vi "GeoData.vi"() -> ()   [LabVIEW 2017] (continued)
city\tID\tFremont County\tH1\n83429\t16043\tIsland park\tID\tFremont County\tH1\n83445\t16043\tSaint anthony\tID\tFremont County\tH1\n83436\t16043\tNewdale\tID\tFremont County\tH1\n83440\t16043\tRexburg\tID\tFremont County\tH1\n83438\t16043\tParker\tID\tFremont County\tH1\n83420\t16043\tAshton\tID\tFremont County\tH1\n83451\t16043\tTeton\tID\tFremont County\tH1\n83433\t16043\tMacks inn\tID\tFremont County\tH1\n83421\t16043\tChester\tID\tFremont County\tH1\n83629\t16045\tHorseshoe bend\tID\tGem County\tH1\n83617\t16045\tEmmett\tID\tGem County\tH1\n83607\t16045\tCaldwell\tID\tGem County\tH1\n83655\t16045\tNew plymouth\tID\tGem County\tH1\n83657\t16045\tOla\tID\tGem County\tH1\n83670\t16045\tSweet\tID\tGem County\tH1\n83636\t16045\tLetha\tID\tGem County\tH1\n83616\t16045\tEagle\tID\tGem County\tH1\n83330\t16047\tGooding\tID\tGooding County\tH1\n83355\t16047\tWendell\tID\tGooding County\tH1\n83338\t16047\tJerome\tID\tGooding County\tH1\n83332\t16047\tHagerman\tID\tGooding County\tH1\n83337\t16047\tHill city\tID\tGooding County\tH1\n83316\t16047\tBuhl\tID\tGooding County\tH1\n83314\t16047\tBliss\tID\tGooding County\tH1\n83352\t16047\tShoshone\tID\tGooding County\tH1\n83549\t16049\tRiggins\tID\tIdaho County\tH1\n83539\t16049\tKooskia\tID\tIdaho County\tH1\n83547\t16049\tPollock\tID\tIdaho County\tH1\n83526\t16049\tFerdinand\tID\tIdaho County\tH1\n83525\t16049\tElk city\tID\tIdaho County\tH1\n83542\t16049\tLucile\tID\tIdaho County\tH1\n83671\t16049\tWarren\tID\tIdaho County\tH1\n83552\t16049\tStites\tID\tIdaho County\tH1\n83522\t16049\tCottonwood\tID\tIdaho County\tH1\n83554\t16049\tWhite bird\tID\tIdaho County\tH1\n83654\t16049\tNew meadows\tID\tIdaho County\tH1\n83530\t16049\tGrangeville\tID\tIdaho County\tH1\n83536\t16049\tKamiah\tID\tIdaho County\tH1\n83533\t16049\tGreencreek\tID\tIdaho County\tH1\n83434\t16051\tMenan\tID\tJefferson County\tH1\n83442\t16051\tRigby\tID\tJefferson County\tH1\n83450\t16051\tTerreton\tID\tJefferson County\tH1\n83443\t16051\tRirie\tID\tJefferson County\tH1\n83425\t16051\tHamer\tID\tJefferson County\tH1\n83444\t16051\tRoberts\tID\tJefferson County\tH1\n83401\t16051\tIdaho falls\tID\tJefferson County\tH1\n83431\t16051\tLewisville\tID\tJefferson County\tH1\n83402\t16051\tIdaho falls\tID\tJefferson County\tH1\n83435\t16051\tMonteview\tID\tJefferson County\tH1\n83325\t16053\tEden\tID\tJerome County\tH1\n83335\t16053\tHazelton\tID\tJerome County\tH1\n83338\t16053\tJerome\tID\tJerome County\tH1\n83301\t16053\tTwin falls\tID\tJerome County\tH1\n83347\t16053\tPaul\tID\tJerome County\tH1\n83810\t16055\tCataldo\tID\tKootenai County\tH1\n83876\t16055\tWorley\tID\tKootenai County\tH1\n83803\t16055\tBayview\tID\tKootenai County\tH1\n83842\t16055\tMedimont\tID\tKootenai County\tH1\n83877\t16055\tPost falls\tID\tKootenai County\tH1\n83815\t16055\tCoeur d alene\tID\tKootenai County\tH1\n83861\t16055\tSaint maries\tID\tKootenai County\tH1\n83869\t16055\tSpirit lake\tID\tKootenai County\tH1\n83816\t16055\tCoeur d alene\tID\tKootenai County\tH1\n83801\t16055\tAthol\tID\tKootenai County\tH1\n83835\t16055\tHayden\tID\tKootenai County\tH1\n83854\t16055\tPost falls\tID\tKootenai County\tH1\n83858\t16055\tRathdrum\tID\tKootenai County\tH1\n83851\t16055\tPlummer\tID\tKootenai County\tH1\n83814\t16055\tCoeur d alene\tID\tKootenai County\tH1\n83833\t16055\tHarrison\tID\tKootenai County\tH1\n83844\t16057\tMoscow\tID\tLatah County\tH1\n83535\t16057\tJuliaetta\tID\tLatah County\tH1\n83843\t16057\tMoscow\tID\tLatah County\tH1\n83823\t16057\tDeary\tID\tLatah County\tH1\n83857\t16057\tPrinceton\tID\tLatah County\tH1\n83834\t16057\tHarvard\tID\tLatah County\tH1\n83806\t16057\tBovill\tID\tLatah County\tH1\n83855\t16057\tPotlatch\tID\tLatah County\tH1\n83824\t16057\tDesmet\tID\tLatah County\tH1\n83872\t16057\tViola\tID\tLatah County\tH1\n83832\t16057\tGenesee\tID\tLatah County\tH1\n83871\t16057\tTroy\tID\tLatah County\tH1\n83537\t16057\tKendrick\tID\tLatah County\tH1\n83253\t16059\tMay\tID\tLemhi County\tH1\n83226\t16059\tChallis\tID\tLemhi County\tH1\n83462\t16059\tCarmen\tID\tLemhi County\tH1\n83469\t16059\tShoup\tID\tLemhi County\tH1\n83468\t16059\tTendoy\tID\tLemhi County\tH1\n83463\t16059\tGibbonsville\tID\tLemhi County\tH1\n83466\t16059\tNorth fork\tID\tLemhi County\tH1\n83235\t16059\tEllis\tID\tLemhi County\tH1\n83467\t16059\tSalmon\tID\tLemhi County\tH1\n83464\t16059\tLeadore\tID\tLemhi County\tH1\n83465\t16059\tLemhi\tID\tLemhi County\tH1\n83229\t16059\tCobalt\tID\tLemhi County\tH1\n83555\t16061\tWinchester\tID\tLewis County\tH1\n83544\t16061\tOrofino\tID\tLewis County\tH1\n83524\t16061\tCuldesac\tID\tLewis County\tH1\n83548\t16061\tReubens\tID\tLewis County\tH1\n83523\t16061\tCraigmont\tID\tLewis County\tH1\n83543\t16061\tNezperce\tID\tLewis County\tH1\n83545\t16061\tPeck\tID\tLewis County\tH1\n83536\t16061\tKamiah\tID\tLewis County\tH1\n83330\t16063\tGooding\tID\tLincoln County\tH1\n83327\t16063\tFairfield\tID\tLincoln County\tH1\n83349\t16063\tRichfield\tID\tLincoln County\tH1\n83324\t16063\tDietrich\tID\tLincoln County\tH1\n83352\t16063\tShoshone\tID\tLincoln County\tH1\n83347\t16063\tPaul\tID\tLincoln County\tH1\n83434\t16065\tMenan\tID\tMadison County\tH1\n83452\t16065\tTetonia\tID\tMadison County\tH1\n83422\t16065\tDriggs\tID\tMadison County\tH1\n83448\t16065\tSugar city\tID\tMadison County\tH1\n83445\t16065\tSaint anthony\tID\tMadison County\tH1\n83436\t16065\tNewdale\tID\tMadison County\tH1\n83440\t16065\tRexburg\tID\tMadison County\tH1\n83460\t16065\tRexburg\tID\tMadison County\tH1\n83451\t16065\tTeton\tID\tMadison County\tH1\n83441\t16065\tRexburg\tID\tMadison County\tH1\n83343\t16067\tMinidoka\tID\tMinidoka County\tH1\n83318\t16067\tBurley\tID\tMinidoka County\tH1\n83350\t16067\tRupert\tID\tMinidoka County\tH1\n83336\t16067\tHeyburn\tID\tMinidoka County\tH1\n83347\t16067\tPaul\tID\tMinidoka County\tH1\n83555\t16069\tWinchester\tID\tNez Perce County\tH1\n83524\t16069\tCuldesac\tID\tNez Perce County\tH1\n83535\t16069\tJuliaetta\tID\tNez Perce County\tH1\n83548\t16069\tReubens\tID\tNez Perce County\tH1\n83501\t16069\tLewiston\tID\tNez Perce County\tH1\n83545\t16069\tPeck\tID\tNez Perce County\tH1\n83540\t16069\tLapwai\tID\tNez Perce County\tH1\n83541\t16069\tLenore\tID\tNez Perce County\tH1\n83832\t16069\tGenesee\tID\tNez Perce County\tH1\n83537\t16069\tKendrick\tID\tNez Perce County\tH1\n83252\t16071\tMalad city\tID\tOneida County\tH1\n83342\t16071\tMalta\tID\tOneida County\tH1\n83243\t16071\tHolbrook\tID\tOneida County\tH1\n83639\t16073\tMarsing\tID\tOwyhee County\tH1\n83641\t16073\tMelba\tID\tOwyhee County\tH1\n83650\t16073\tMurphy\tID\tOwyhee County\tH1\n83604\t16073\tBruneau\tID\tOwyhee County\tH1\n83627\t16073\tHammett\tID\tOwyhee County\tH1\n83628\t16073\tHomedale\tID\tOwyhee County\tH1\n83624\t16073\tGrand view\tID\tOwyhee County\tH1\n83302\t16073\tRogerson\tID\tOwyhee County\tH1\n83619\t16075\tFruitland\tID\tPayette County\tH1\n83660\t16075\tParma\tID\tPayette County\tH1\n83607\t16075\tCaldwell\tID\tPayette County\tH1\n83655\t16075\tNew plymouth\tID\tPayette County\tH1\n83661\t16075\tPayette\tID\tPayette County\tH1\n83204\t16077\tPocatello\tID\tPower County\tH1\n83271\t16077\tRockland\tID\tPower County\tH1\n83211\t16077\tAmerican falls\tID\tPower County\tH1\n83212\t16077\tArbon\tID\tPower County\tH1\n83830\t16079\tFernwood\tID\tShoshone County\tH1\n83849\t16079\tOsburn\tID\tShoshone County\tH1\n83810\t16079\tCataldo\tID\tShoshone County\tH1\n83802\t16079\tAvery\tID\tShoshone County\tH1\n83868\t16079\tSmelterville\tID\tShoshone County\tH1\n83850\t16079\tPinehurst\tID\tShoshone County\tH1\n83861\t16079\tSaint maries\tID\tShoshone County\tH1\n83873\t16079\tWallace\tID\tShoshone County\tH1\n83839\t16079\tKingston\tID\tShoshone County\tH1\n83846\t16079\tMullan\tID\tShoshone County\tH1\n83837\t16079\tKellogg\tID\tShoshone County\tH1\n83867\t16079\tSilverton\tID\tShoshone County\tH1\n83808\t16079\tCalder\tID\tShoshone County\tH1\n83812\t16079\tClarkia\tID\tShoshone County\tH1\n83874\t16079\tMurray\tID\tShoshone County\tH1\n83424\t16081\tFelt\tID\tTeton County\tH1\n83452\t16081\tTetonia\tID\tTeton County\tH1\n83422\t16081\tDriggs\tID\tTeton County\tH1\n83455\t16081\tVictor\tID\tTeton County\tH1\n83436\t16081\tNewdale\tID\tTeton County\tH1\n83303\t16083\tTwin falls\tID\tTwin Falls County\tH1\n83328\t16083\tFiler\tID\tTwin Falls County\tH1\n83332\t16083\tHagerman\tID\tTwin Falls County\tH1\n83344\t16083\tMurtaugh\tID\tTwin Falls County\tH1\n83301\t16083\tTwin falls\tID\tTwin Falls County\tH1\n83321\t16083\tCastleford\tID\tTwin Falls County\tH1\n83316\t16083\tBuhl\tID\tTwin Falls County\tH1\n83341\t16083\tKimberly\tID\tTwin Falls County\tH1\n83334\t16083\tHansen\tID\tTwin Falls County\tH1\n83302\t16083\tRogerson\tID\tTwin Falls County\tH1\n83638\t16085\tMccall\tID\tValley County\tH1\n83615\t16085\tDonnelly\tID\tValley County\tH1\n83677\t16085\tYellow pine\tID\tValley County\tH1\n83611\t16085\tCascade\tID\tValley County\tH1\n83635\t16085\tLake fork\tID\tValley County\tH1\n83632\t16087\tIndian valley\tID\tWashington County\tH1\n83645\t16087\tMidvale\tID\tWashington County\tH1\n83610\t16087\tCambridge\tID\tWashington County\tH1\n83672\t16087\tWeiser\tID\tWashington County\tH1\n83661\t16087\tPayette\tID\tWashington County\tH1\n62301\t17001\tQuincy\tIL\tAdams County\tH1\n62306\t17001\tQuincy\tIL\tAdams County\tH1\n62379\t17001\tWarsaw\tIL\tAdams County\tH1\n62376\t17001\tUrsa\tIL\tAdams County\tH1\n62316\t17001\tBowen\tIL\tAdams County\tH1\n62314\t17001\tBaylis\tIL\tAdams County\tH1\n62365\t17001\tPlainville\tIL\tAdams County\tH1\n62320\t17001\tCamp point\tIL\tAdams County\tH1\n62305\t17001\tQuincy\tIL\tAdams County\tH1\n62351\t17001\tMendon\tIL\tAdams County\tH1\n62380\t17001\tWest point\tIL\tAdams County\tH1\n62324\t17001\tClayton\tIL\tAdams County\tH1\n62343\t17001\tHull\tIL\tAdams County\tH1\n62360\t17001\tPayson\tIL\tAdams County\tH1\n62312\t17001\tBarry\tIL\tAdams County\tH1\n62373\t17001\tSutter\tIL\tAdams County\tH1\n62347\t17001\tLiberty\tIL\tAdams County\tH1\n62346\t17001\tLa prairie\tIL\tAdams County\tH1\n62311\t17001\tAugusta\tIL\tAdams County\tH1\n62359\t17001\tPaloma\tIL\tAdams County\tH1\n62348\t17001\tLima\tIL\tAdams County\tH1\n62339\t17001\tGolden\tIL\tAdams County\tH1\n62349\t17001\tLoraine\tIL\tAdams County\tH1\n62338\t17001\tFowler\tIL\tAdams County\tH1\n62325\t17001\tCoatsburg\tIL\tAdams County\tH1\n62914\t17003\tCairo\tIL\tAlexander County\tH1\n62962\t17003\tMiller city\tIL\tAlexander County\tH1\n62952\t17003\tJonesboro\tIL\tAlexander County\tH1\n62957\t17003\tMc clure\tIL\tAlexander County\tH1\n62969\t17003\tOlive branch\tIL\tAlexander County\tH1\n62990\t17003\tThebes\tIL\tAlexander County\tH1\n62992\t17003\tUllin\tIL\tAlexander County\tH1\n62993\t17003\tUnity\tIL\tAlexander County\tH1\n62988\t17003\tTamms\tIL\tAlexander County\tH1\n62249\t17005\tHighland\tIL\tBond County\tH1\n62231\t17005\tCarlyle\tIL\tBond County\tH1\n62275\t17005\tPocahontas\tIL\tBond County\tH1\n62019\t17005\tDonnellson\tIL\tBond County\tH1\n62253\t17005\tKeyesport\tIL\tBond County\tH1\n62262\t17005\tMulberry grove\tIL\tBond County\tH1\n62017\t17005\tCoffeen\tIL\tBond County\tH1\n62086\t17005\tSorento\tIL\tBond County\tH1\n62074\t17005\tNew douglas\tIL\tBond County\tH1\n62284\t17005\tSmithboro\tIL\tBond County\tH1\n62246\t17005\tGreenville\tIL\tBond County\tH1\n61114\t17007\tRockford\tIL\tBoone County\tH1\n60152\t17007\tMarengo\tIL\tBoone County\tH1\n61011\t17007\tCaledonia\tIL\tBoone County\tH1\n61012\t17007\tCapron\tIL\tBoone County\tH1\n61008\t17007\tBelvidere\tIL\tBoone County\tH1\n61073\t17007\tRoscoe\tIL\tBoone County\tH1\n61080\t17007\tSouth beloit\tIL\tBoone County\tH1\n61038\t17007\tGarden prairie\tIL\tBoone County\tH1\n61111\t17007\tLoves park\tIL\tBoone County\tH1\n60033\t17007\tHarvard\tIL\tBoone County\tH1\n60145\t17007\tKingston\tIL\tBoone County\tH1\n61065\t17007\tPoplar grove\tIL\tBoone County\tH1\n61107\t17007\tRockford\tIL\tBoone County\tH1\n61108\t17007\tRockford\tIL\tBoone County\tH1\n60135\t17007\tGenoa\tIL\tBoone County\tH1\n60146\t17007\tKirkland\tIL\tBoone County\tH1\n61016\t17007\tCherry valley\tIL\tBoone County\tH1\n62375\t17009\tTimewell\tIL\tBrown County\tH1\n62314\t17009\tBaylis\tIL\tBrown County\tH1\n62353\t17009\tMount sterling\tIL\tBrown County\tH1\n62378\t17009\tVersailles\tIL\tBrown County\tH1\n61560\t17011\tPutnam\tIL\tBureau County\tH1\n61338\t17011\tManlius\tIL\tBureau County\tH1\n61421\t17011\tBradford\tIL\tBureau County\tH1\n61337\t17011\tMalden\tIL\tBureau County\tH1\n61349\t17011\tOhio\tIL\tBureau County\tH1\n61314\t17011\tBuda\tIL\tBureau County\tH1\n61443\t17011\tKewanee\tIL\tBureau County\tH1\n61342\t17011\tMendota\tIL\tBureau County\tH1\n61379\t17011\tWyanet\tIL\tBureau County\tH1\n61312\t17011\tArlington\tIL\tBureau County\tH1\n61344\t17011\tMineral\tIL\tBureau County\tH1\n61346\t17011\tNew bedford\tIL\tBureau County\tH1\n61283\t17011\tTampico\tIL\tBureau County\tH1\n61356\t17011\tPrinceton\tIL\tBureau County\tH1\n61374\t17011\tVan orin\tIL\tBureau County\tH1\n61243\t17011\tDeer grove\tIL\tBureau County\tH1\n61354\t17011\tPeru\tIL\tBureau County\tH1\n61362\t17011\tSpring valley\tIL\tBureau County\tH1\n61368\t17011\tTiskilwa\tIL\tBureau County\tH1\n61376\t17011\tWalnut\tIL\tBureau County\tH1\n61315\t17011\tBureau\tIL\tBureau County\tH1\n61361\t17011\tSheffield\tIL\tBureau County\tH1\n61345\t17011\tNeponset\tIL\tBureau County\tH1\n61320\t17011\tDalzell\tIL\tBureau County\tH1\n61317\t17011\tCherry\tIL\tBureau County\tH1\n61329\t17011\tLadd\tIL\tBureau County\tH1\n61330\t17011\tLa moille\tIL\tBureau County\tH1\n61359\t17011\tSeatonville\tIL\tBureau County\tH1\n61323\t17011\tDover\tIL\tBureau County\tH1\n61328\t17011\tKasbeer\tIL\tBureau County\tH1\n61234\t17011\tAnnawan\tIL\tBureau County\tH1\n61322\t17011\tDepue\tIL\tBureau County\tH1\n62047\t17013\tHardin\tIL\tCalhoun County\tH1\n62070\t17013\tMozier\tIL\tCalhoun County\tH1\n62053\t17013\tKampsville\tIL\tCalhoun County\tH1\n62006\t17013\tBatchtown\tIL\tCalhoun County\tH1\n62045\t17013\tHamburg\tIL\tCalhoun County\tH1\n62036\t17013\tGolden eagle\tIL\tCalhoun County\tH1\n62355\t17013\tNebo\tIL\tCalhoun County\tH1\n62065\t17013\tMichael\tIL\tCalhoun County\tH1\n62013\t17013\tBrussels\tIL\tCalhoun County\tH1\n61053\t17015\tMount carroll\tIL\tCarroll County\tH1\n61062\t17015\tPearl city\tIL\tCarroll County\tH1\n61285\t17015\tThomson\tIL\tCarroll County\tH1\n61051\t17015\tMilledgeville\tIL\tCarroll County\tH1\n61064\t17015\tPolo\tIL\tCarroll County\tH1\n61252\t17015\tFulton\tIL\tCarroll County\tH1\n61028\t17015\tElizabeth\tIL\tCarroll County\tH1\n61074\t17015\tSavanna\tIL\tCarroll County\tH1\n61270\t17015\tMorrison\tIL\tCarroll County\tH1\n61046\t17015\tLanark\tIL\tCarroll County\tH1\n61078\t17015\tShannon\tIL\tCarroll County\tH1\n61014\t17015\tChadwick\tIL\tCarroll County\tH1\n62627\t17017\tChandlerville\tIL\tCass County\tH1\n62665\t17017\tMeredosia\tIL\tCass County\tH1\n62677\t17017\tPleasant plains\tIL\tCass County\tH1\n62612\t17017\tAshland\tIL\tCass County\tH1\n62618\t17017\tBeardstown\tIL\tCass County\tH1\n62691\t17017\tVirginia\tIL\tCass County\tH1\n62673\t17017\tOakford\tIL\tCass County\tH1\n62675\t17017\tPetersburg\tIL\tCass County\tH1\n62611\t17017\tArenzville\tIL\tCass County\tH1\n62622\t17017\tBluff springs\tIL\tCass County\tH1\n61864\t17019\tPhilo\tIL\tChampaign County\tH1\n60949\t17019\tLudlow\tIL\tChampaign County\tH1\n60957\t17019\tPaxton\tIL\tChampaign County\tH1\n61802\t17019\tUrbana\tIL\tChampaign County\tH1\n61859\t17019\tOgden\tIL\tChampaign County\tH1\n61862\t17019\tPenfield\tIL\tChampaign County\tH1\n61872\t17019\tSadorus\tIL\tChampaign County\tH1\n61852\t17019\tLongview\tIL\tChampaign County\tH1\n61856\t17019\tMonticello\tIL\tChampaign County\tH1\n61878\t17019\tThomasboro\tIL\tChampaign County\tH1\n61843\t17019\tFisher\tIL\tChampaign County\tH1\n61884\t17019\tWhite heath\tIL\tChampaign County\tH1\n61851\t17019\tIvesdale\tIL\tChampaign County\tH1\n60936\t17019\tGibson city\tIL\tChampaign County\tH1\n61956\t17019\tVilla grove\tIL\tChampaign County\tH1\n61863\t17019\tPesotum\tIL\tChampaign County\tH1\n60960\t17019\tRankin\tIL\tChampaign County\tH1\n61849\t17019\tHomer\tIL\tChampaign County\tH1\n61880\t17019\tTolono\tIL\tChampaign County\tH1\n61866\t17019\tRantoul\tIL\tChampaign County\tH1\n61847\t17019\tGifford\tIL\tChampaign County\tH1\n61825\t17019\tChampaign\tIL\tChampaign County\tH1\n61822\t17019\tChampaign\tIL\tChampaign County\tH1\n61815\t17019\tBondville\tIL\tChampaign County\tH1\n61853\t17019\tMahomet\tIL\tChampaign County\tH1\n61953\t17019\tTuscola\tIL\tChampaign County\tH1\n61854\t17019\tMansfield\tIL\tChampaign County\tH1\n61810\t17019\tAllerton\tIL\tChampaign County\tH1\n61801\t17019\tUrbana\tIL\tChampaign County\tH1\n61821\t17019\tChampaign\tIL\tChampaign County\tH1\n61826\t17019\tChampaign\tIL\tChampaign County\tH1\n61873\t17019\tSaint joseph\tIL\tChampaign County\tH1\n61840\t17019\tDewey\tIL\tChampaign County\tH1\n61871\t17019\tRoyal\tIL\tChampaign County\tH1\n61845\t17019\tFoosland\tIL\tChampaign County\tH1\n61824\t17019\tChampaign\tIL\tChampaign County\tH1\n61820\t17019\tChampaign\tIL\tChampaign County\tH1\n61874\t17019\tSavoy\tIL\tChampaign County\tH1\n61875\t17019\tSeymour\tIL\tChampaign County\tH1\n61877\t17019\tSidney\tIL\tChampaign County\tH1\n61816\t17019\tBroadlands\tIL\tChampaign County\tH1\n61803\t17019\tUrbana\tIL\tChampaign County\tH1\n62545\t17021\tMechanicsburg\tIL\tChristian County\tH1\n62510\t17021\tAssumption\tIL\tChristian County\tH1\n62556\t17021\tPalmer\tIL\tChristian County\tH1\n62547\t17021\tMount auburn\tIL\tChristian County\tH1\n62555\t17021\tOwaneco\tIL\tChristian County\tH1\n62083\t17021\tRosamond\tIL\tChristian County\tH1\n62558\t17021\tPawnee\tIL\tChristian County\tH1\n62557\t17021\tPana\tIL\tChristian County\tH1\n62546\t17021\tMorrisonville\tIL\tChristian County\tH1\n62567\t17021\tStonington\tIL\tChristian County\tH1\n62568\t17021\tTaylorville\tIL\tChristian County\tH1\n62075\t17021\tNokomis\tIL\tChristian County\tH1\n62540\t17021\tKincaid\tIL\tChristian County\tH1\n62531\t17021\tEdinburg\tIL\tChristian County\tH1\n62538\t17021\tHarvel\tIL\tChristian County\tH1\n62513\t17021\tBlue mound\tIL\tChristian County\tH1\n62563\t17021\tRochester\tIL\tChristian County\tH1\n62550\t17021\tMoweaqua\tIL\tChristian County\tH1\n62570\t17021\tTovey\tIL\tChristian County\tH1\n62517\t17021\tBulpitt\tIL\tChristian County\tH1\n62478\t17023\tWest york\tIL\tClark County\tH1\n61933\t17023\tKansas\tIL\tClark County\tH1\n61944\t17023\tParis\tIL\tClark County\tH1\n62420\t17023\tCasey\tIL\tClark County\tH1\n62441\t17023\tMarshall\tIL\tClark County\tH1\n62481\t17023\tYale\tIL\tClark County\tH1\n61912\t17023\tAshmore\tIL\tClark County\tH1\n62413\t17023\tAnnapolis\tIL\tClark County\tH1\n62449\t17023\tOblong\tIL\tClark County\tH1\n62442\t17023\tMartinsville\tIL\tClark County\tH1\n62474\t17023\tWestfield\tIL\tClark County\tH1\n62423\t17023\tDennison\tIL\tClark County\tH1\n62477\t17023\tWest union\tIL\tClark County\tH1\n62448\t17025\tNewton\tIL\tClay County\tH1\n62426\t17025\tEdgewood\tIL\tClay County\tH1\n62858\t17025\tLouisville\tIL\tClay County\tH1\n62899\t17025\tXenia\tIL\tClay County\tH1\n62838\t17025\tFarina\tIL\tClay County\tH1\n62839\t17025\tFlora\tIL\tClay County\tH1\n62868\t17025\tNoble\tIL\tClay County\tH1\n62879\t17025\tSailor springs\tIL\tClay County\tH1\n62443\t17025\tMason\tIL\tClay County\tH1\n62424\t17025\tDieterich\tIL\tClay County\tH1\n62824\t17025\tClay city\tIL\tClay County\tH1\n62854\t17025\tKinmundy\tIL\tClay County\tH1\n62434\t17025\tIngraham\tIL\tClay County\tH1\n62249\t17027\tHighland\tIL\tClinton County\tH1\n62231\t17027\tCarlyle\tIL\tClinton County\tH1\n62275\t17027\tPocahontas\tIL\tClinton County\tH1\n62219\t17027\tBeckemeyer\tIL\tClinton County\tH1\n62882\t17027\tSandoval\tIL\tClinton County\tH1\n62253\t17027\tKeyesport\tIL\tClinton County\tH1\n62252\t17027\tHuey\tIL\tClinton County\tH1\n62250\t17027\tHoffman\tIL\tClinton County\tH1\n62266\t17027\tNew memphis\tIL\tClinton County\tH1\n62215\t17027\tAlbers\tIL\tClinton County\tH1\n62801\t17027\tCentralia\tIL\tClinton County\tH1\n62875\t17027\tPatoka\tIL\tClinton County\tH1\n62216\t17027\tAviston\tIL\tClinton County\tH1\n62230\t17027\tBreese\tIL\tClinton County\tH1\n62265\t17027\tNew baden\tIL\tClinton County\tH1\n62218\t17027\tBartelso\tIL\tClinton County\tH1\n62245\t17027\tGermantown\tIL\tClinton County\tH1\n62246\t17027\tGreenville\tIL\tClinton County\tH1\n62258\t17027\tMascoutah\tIL\tClinton County\tH1\n62293\t17027\tTrenton\tIL\tClinton County\tH1\n62447\t17029\tNeoga\tIL\tColes County\tH1\n61920\t17029\tCharleston\tIL\tColes County\tH1\n62469\t17029\tTrilla\tIL\tColes County\tH1\n62440\t17029\tLerna\tIL\tColes County\tH1\n61931\t17029\tHumboldt\tIL\tColes County\tH1\n62420\t17029\tCasey\tIL\tColes County\tH1\n61943\t17029\tOakland\tIL\tColes County\tH1\n61911\t17029\tArthur\tIL\tColes County\tH1\n61930\t17029\tHindsboro\tIL\tColes County\tH1\n61912\t17029\tAshmore\tIL\tColes County\tH1\n61910\t17029\tArcola\tIL\tColes County\tH1\n61938\t17029\tMattoon\tIL\tColes County\tH1\n61951\t17029\tSullivan\tIL\tColes County\tH1\n61928\t17029\tGays\tIL\tColes County\tH1\n62474\t17029\tWestfield\tIL\tColes County\tH1\n60067\t17031\tPalatine\tIL\tCook County\tH1\n60056\t17031\tMount prospect\tIL\tCook County\tH1\n60029\t17031\tGolf\tIL\tCook County\tH1\n60305\t17031\tRiver forest\tIL\tCook County\tH1\n60417\t17031\tCrete\tIL\tCook County\tH1\n60422\t17031\tFlossmoor\tIL\tCook County\tH1\n60462\t17031\tOrland park\tIL\tCook County\tH1\n60455\t17031\tBridgeview\tIL\tCook County\tH1\n60456\t17031\tHometown\tIL\tCook County\tH1\n60463\t17031\tPalos heights\tIL\tCook County\tH1\n60525\t17031\tLa grange\tIL\tCook County\tH1\n60162\t17031\tHillside\tIL\tCook County\tH1\n60619\t17031\tChicago\tIL\tCook County\tH1\n60654\t17031\tChicago\tIL\tCook County\tH1\n60632\t17031\tChicago\tIL\tCook County\tH1\n60682\t17031\tChicago\tIL\tCook County\tH1\n60689\t17031\tChicago\tIL\tCook County\tH1\n60684\t17031\tChicago\tIL\tCook County\tH1\n60669\t17031\tChicago\tIL\tCook County\tH1\n60068\t17031\tPark ridge\tIL\tCook County\tH1\n60090\t17031\tWheeling\tIL\tCook County\tH1\n60091\t17031\tWilmette\tIL\tCook County\tH1\n60089\t17031\tBuffalo grove\tIL\tCook County\tH1\n60053\t17031\tMorton grove\tIL\tCook County\tH1\n60203\t17031\tEvanston\tIL\tCook County\tH1\n60192\t17031\tHoffman estates\tIL\tCook County\tH1\n60402\t17031\tBerwyn\tIL\tCook County\tH1\n60303\t17031\tOak park\tIL\tCook County\tH1\n60172\t17031\tRoselle\tIL\tCook County\tH1\n60195\t17031\tSchaumburg\tIL\tCook County\tH1\n60176\t17031\tSchiller park\tIL\tCook County\tH1\n60439\t17031\tLemont\tIL\tCook County\tH1\n60423\t17031\tFrankfort\tIL\tCook County\tH1\n60457\t17031\tHickory hills\tIL\tCook County\tH1\n60523\t17031\tOak brook\tIL\tCook County\tH1\n60480\t17031\tWillow springs\tIL\tCook County\tH1\n60163\t17031\tBerkeley\tIL\tCook County\tH1\n60558\t17031\tWestern springs\tIL\tCook County\tH1\n60615\t17031\tChicago\tIL\tCook County\tH1\n60616\t17031\tChicago\tIL\tCook County\tH1\n60608\t17031\tChicago\tIL\tCook County\tH1\n60620\t17031\tChicago\tIL\tCook County\tH1\n60651\t17031\tChicago\tIL\tCook County\tH1\n60659\t17031\tChicago\tIL\tCook County\tH1\n60706\t17031\tHarwood heights\tIL\tCook County\tH1\n60653\t17031\tChicago\tIL\tCook County\tH1\n60639\t17031\tChicago\tIL\tCook County\tH1\n60624\t17031\tChicago\tIL\tCook County\tH1\n60647\t17031\tChicago\tIL\tCook County\tH1\n60011\t17031\tBarrington\tIL\tCook County\tH1\n60690\t17031\tChicago\tIL\tCook County\tH1\n60006\t17031\tArlington heights\tIL\tCook County\tH1\n60695\t17031\tChicago\tIL\tCook County\tH1\n60687\t17031\tChicago\tIL\tCook County\tH1\n60678\t17031\tChicago\tIL\tCook County\tH1\n60685\t17031\tChicago\tIL\tCook County\tH1\n60196\t17031\tSchaumburg\tIL\tCook County\tH1\n60070\t17031\tProspect heights\tIL\tCook County\tH1\n60026\t17031\tGlenview\tIL\tCook County\tH1\n60008\t17031\tRolling meadows\tIL\tCook County\tH1\n60301\t17031\tOak park\tIL\tCook County\tH1\n60411\t17031\tChicago heights\tIL\tCook County\tH1\n60415\t17031\tChicago ridge\tIL\tCook County\tH1\n60169\t17031\tHoffman estates\tIL\tCook County\tH1\n60438\t17031\tLansing\tIL\tCook County\tH1\n60428\t17031\tMarkham\tIL\tCook County\tH1\n60458\t17031\tJustice\tIL\tCook County\tH1\n60425\t17031\tGlenwood\tIL\tCook County\tH1\n60418\t17031\tCrestwood\tIL\tCook County\tH1\n60513\t17031\tBrookfield\tIL\tCook County\tH1\n60501\t17031\tSummit argo\tIL\tCook County\tH1\n60103\t17031\tBartlett\tIL\tCook County\tH1\n60102\t17031\tAlgonquin\tIL\tCook County\tH1\n60154\t17031\tWestchester\tIL\tCook County\tH1\n60155\t17031\tBroadview\tIL\tCook County\tH1\n60609\t17031\tChicago\tIL\tCook County\tH1\n60803\t17031\tAlsip\tIL\tCook County\tH1\n60675\t17031\tChicago\tIL\tCook County\tH1\n60633\t17031\tChicago\tIL\tCook County\tH1\n60634\t17031\tChicago\tIL\tCook County\tH1\n60645\t17031\tChicago\tIL\tCook County\tH1\n60208\t17031\tEvanston\tIL\tCook County\tH1\n60699\t17031\tChicago\tIL\tCook County\tH1\n60038\t17031\tPalatine\tIL\tCook County\tH1\n60668\t17031\tChicago\tIL\tCook County\tH1\n60701\t17031\tChicago\tIL\tCook County\tH1\n60062\t17031\tNorthbrook\tIL\tCook County\tH1\n60016\t17031\tDes plaines\tIL\tCook County\tH1\n60015\t17031\tDeerfield\tIL\tCook County\tH1\n60018\t17031\tDes plaines\tIL\tCook County\tH1\n60043\t17031\tKenilworth\tIL\tCook County\tH1\n60409\t17031\tCalumet city\tIL\tCook County\tH1\n60443\t17031\tMatteson\tIL\tCook County\tH1\n60465\t17031\tPalos hills\tIL\tCook County\tH1\n60469\t17031\tPosen\tIL\tCook County\tH1\n60471\t17031\tRichton park\tIL\tCook County\tH1\n60131\t17031\tFranklin park\tIL\tCook County\tH1\n60153\t17031\tMaywood\tIL\tCook County\tH1\n60613\t17031\tChicago\tIL\tCook County\tH1\n60622\t17031\tChicago\tIL\tCook County\tH1\n60804\t17031\tCicero\tIL\tCook County\tH1\n60649\t17031\tChicago\tIL\tCook County\tH1\n60652\t17031\tChicago\tIL\tCook County\tH1\n60631\t17031\tChicago\tIL\tCook County\tH1\n60640\t17031\tChicago\tIL\tCook County\tH1\n60626\t17031\tChicago\tIL\tCook County\tH1\n60630\t17031\tChicago\tIL\tCook County\tH1\n60636\t17031\tChicago\tIL\tCook County\tH1\n60643\t17031\tChicago\tIL\tCook County\tH1\n60499\t17031\tBedford park\tIL\tCook County\tH1\n60082\t17031\tTechny\tIL\tCook County\tH1\n60076\t17031\tSkokie\tIL\tCook County\tH1\n60202\t17031\tEvanston\tIL\tCook County\tH1\n60093\t17031\tWinnetka\tIL\tCook County\tH1\n60005\t17031\tArlington heights\tIL\tCook County\tH1\n60194\t17031\tSchaumburg\tIL\tCook County\tH1\n60302\t17031\tOak park\tIL\tCook County\tH1\n60164\t17031\tMelrose park\tIL\tCook County\tH1\n60448\t17031\tMokena\tIL\tCook County\tH1\n60453\t17031\tOak lawn\tIL\tCook County\tH1\n60459\t17031\tBurbank\tIL\tCook County\tH1\n60487\t17031\tTinley park\tIL\tCook County\tH1\n60466\t17031\tPark forest\tIL\tCook County\tH1\n60120\t17031\tElgin\tIL\tCook County\tH1\n60546\t17031\tRiverside\tIL\tCook County\tH1\n60605\t17031\tChicago\tIL\tCook County\tH1\n60607\t17031\tChicago\tIL\tCook County\tH1\n60612\t17031\tChicago\tIL\tCook County\tH1\n60621\t17031\tChicago\tIL\tCook County\tH1\n60657\t17031\tChicago\tIL\tCook County\tH1\n60655\t17031\tChicago\tIL\tCook County\tH1\n60629\t17031\tChicago\tIL\tCook County\tH1\n60637\t17031\tChicago\tIL\tCook County\tH1\n60641\t17031\tChicago\tIL\tCook County\tH1\n60625\t17031\tChicago\tIL\tCook County\tH1\n60646\t17031\tChicago\tIL\tCook County\tH1\n60602\t17031\tChicago\tIL\tCook County\tH1\n60159\t17031\tSchaumburg\tIL\tCook County\tH1\n60673\t17031\tChicago\tIL\tCook County\tH1\n60694\t17031\tChicago\tIL\tCook County\tH1\n60095\t17031\tPalatine\tIL\tCook County\tH1\n60055\t17031\tPalatine\tIL\tCook County\tH1\n60670\t17031\tChicago\tIL\tCook County\tH1\n60077\t17031\tSkokie\tIL\tCook County\tH1\n60201\t17031\tEvanston\tIL\tCook County\tH1\n60204\t17031\tEvanston\tIL\tCook County\tH1\n60010\t17031\tBarrington\tIL\tCook County\tH1\n60007\t17031\tElk grove village\tIL\tCook County\tH1\n60304\t17031\tOak park\tIL\tCook County\tH1\n60419\t17031\tDolton\tIL\tCook County\tH1\n60445\t17031\tMidlothian\tIL\tCook County\tH1\n60452\t17031\tOak forest\tIL\tCook County\tH1\n60521\t17031\tHinsdale\tIL\tCook County\tH1\n60527\t17031\tWillowbrook\tIL\tCook County\tH1\n60472\t17031\tRobbins\tIL\tCook County\tH1\n60141\t17031\tHines\tIL\tCook County\tH1\n60130\t17031\tForest park\tIL\tCook County\tH1\n60107\t17031\tStreamwood\tIL\tCook County\tH1\n60160\t17031\tMelrose park\tIL\tCook County\tH1\n60610\t17031\tChicago\tIL\tCook County\tH1\n60603\t17031\tChicago\tIL\tCook County\tH1\n60827\t17031\tRiverdale\tIL\tCook County\tH1\n60714\t17031\tNiles\tIL\tCook County\tH1\n60656\t17031\tChicago\tIL\tCook County\tH1\n60476\t17031\tThornton\tIL\tCook County\tH1\n60078\t17031\tPalatine\tIL\tCook County\tH1\n60666\t17031\tChicago\tIL\tCook County\tH1\n60454\t17031\tOak lawn\tIL\tCook County\tH1\n60065\t17031\tNorthbrook\tIL\tCook County\tH1\n60697\t17031\tChicago\tIL\tCook County\tH1\n60074\t17031\tPalatine\tIL\tCook County\tH1\n60022\t17031\tGlencoe\tIL\tCook County\tH1\n60004\t17031\tArlington heights\tIL\tCook County\tH1\n60025\t17031\tGlenview\tIL\tCook County\tH1\n60193\t17031\tSchaumburg\tIL\tCook County\tH1\n60173\t17031\tSchaumburg\tIL\tCook County\tH1\n60406\t17031\tBlue island\tIL\tCook County\tH1\n60412\t17031\tChicago heights\tIL\tCook County\tH1\n60449\t17031\tMonee\tIL\tCook County\tH1\n60426\t17031\tHarvey\tIL\tCook County\tH1\n60430\t17031\tHomewood\tIL\tCook County\tH1\n60477\t17031\tTinley park\tIL\tCook County\tH1\n60482\t17031\tWorth\tIL\tCook County\tH1\n60473\t17031\tSouth holland\tIL\tCook County\tH1\n60478\t17031\tCountry club hills\tIL\tCook County\tH1\n60526\t17031\tLa grange park\tIL\tCook County\tH1\n60484\t17031\tUniversity park\tIL\tCook County\tH1\n60534\t17031\tLyons\tIL\tCook County\tH1\n60618\t17031\tChicago\tIL\tCook County\tH1\n60604\t17031\tChicago\tIL\tCook County\tH1\n60606\t17031\tChicago\tIL\tCook County\tH1\n60617\t17031\tChicago\tIL\tCook County\tH1\n60660\t17031\tChicago\tIL\tCook County\tH1\n60661\t17031\tChicago\tIL\tCook County\tH1\n60712\t17031\tLincolnwood\tIL\tCook County\tH1\n60805\t17031\tEvergreen park\tIL\tCook County\tH1\n60674\t17031\tChicago\tIL\tCook County\tH1\n60628\t17031\tChicago\tIL\tCook County\tH1\n60623\t17031\tChicago\tIL\tCook County\tH1\n60677\t17031\tChicago\tIL\tCook County\tH1\n60681\t17031\tChicago\tIL\tCook County\tH1\n60688\t17031\tChicago\tIL\tCook County\tH1\n60017\t17031\tDes plaines\tIL\tCook County\tH1\n60171\t17031\tRiver grove\tIL\tCook County\tH1\n60165\t17031\tStone park\tIL\tCook County\tH1\n60429\t17031\tHazel crest\tIL\tCook County\tH1\n60461\t17031\tOlympia fields\tIL\tCook County\tH1\n60491\t17031\tHomer glen\tIL\tCook County\tH1\n60464\t17031\tPalos park\tIL\tCook County\tH1\n60467\t17031\tOrland park\tIL\tCook County\tH1\n60475\t17031\tSteger\tIL\tCook County\tH1\n60126\t17031\tElmhurst\tIL\tCook County\tH1\n60133\t17031\tHanover park\tIL\tCook County\tH1\n60104\t17031\tBellwood\tIL\tCook County\tH1\n60118\t17031\tDundee\tIL\tCook County\tH1\n60611\t17031\tChicago\tIL\tCook County\tH1\n60614\t17031\tChicago\tIL\tCook County\tH1\n60707\t17031\tElmwood park\tIL\tCook County\tH1\n60638\t17031\tChicago\tIL\tCook County\tH1\n60642\t17031\tChicago\tIL\tCook County\tH1\n60644\t17031\tChicago\tIL\tCook County\tH1\n60601\t17031\tChicago\tIL\tCook County\tH1\n60161\t17031\tMelrose park\tIL\tCook County\tH1\n60686\t17031\tChicago\tIL\tCook County\tH1\n60009\t17031\tElk grove village\tIL\tCook County\tH1\n60693\t17031\tChicago\tIL\tCook County\tH1\n60168\t17031\tSchaumburg\tIL\tCook County\tH1\n60179\t17031\tHoffman estates\tIL\tCook County\tH1\n62466\t17033\tSumner\tIL\tCrawford County\tH1\n62478\t17033\tWest york\tIL\tCrawford County\tH1\n62433\t17033\tHutsonville\tIL\tCrawford County\tH1\n62454\t17033\tRobinson\tIL\tCrawford County\tH1\n62451\t17033\tPalestine\tIL\tCrawford County\tH1\n62421\t17033\tClaremont\tIL\tCrawford County\tH1\n62464\t17033\tStoy\tIL\tCrawford County\tH1\n62413\t17033\tAnnapolis\tIL\tCrawford County\tH1\n62427\t17033\tFlat rock\tIL\tCrawford County\tH1\n62449\t17033\tOblong\tIL\tCrawford County\tH1\n62442\t17033\tMartinsville\tIL\tCrawford County\tH1\n62447\t17035\tNeoga\tIL\tCumberland County\tH1\n61920\t17035\tCharleston\tIL\tCumberland County\tH1\n62469\t17035\tTrilla\tIL\tCumberland County\tH1\n62440\t17035\tLerna\tIL\tCumberland County\tH1\n62445\t17035\tMontrose\tIL\tCumberland County\tH1\n62420\t17035\tCasey\tIL\tCumberland County\tH1\n62428\t17035\tGreenup\tIL\tCumberland County\tH1\n62468\t17035\tToledo\tIL\tCumberland County\tH1\n62432\t17035\tHidalgo\tIL\tCumberland County\tH1\n62462\t17035\tSigel\tIL\tCumberland County\tH1\n62436\t17035\tJewett\tIL\tCumberland County\tH1\n61938\t17035\tMattoon\tIL\tCumberland County\tH1\n62467\t17035\tTeutopolis\tIL\tCumberland County\tH1\n60152\t17037\tMarengo\tIL\tDeKalb County\tH1\n60553\t17037\tSteward\tIL\tDeKalb County\tH1\n60112\t17037\tCortland\tIL\tDeKalb County\tH1\n60552\t17037\tSomonauk\tIL\tDeKalb County\tH1\n60548\t17037\tSandwich\tIL\tDeKalb County\tH1\n61068\t17037\tRochelle\tIL\tDeKalb County\tH1\n60178\t17037\tSycamore\tIL\tDeKalb County\tH1\n60531\t17037\tLeland\tIL\tDeKalb County\tH1\n60111\t17037\tClare\tIL\tDeKalb County\tH1\n60115\t17037\tDekalb\tIL\tDeKalb County\tH1\n61052\t17037\tMonroe center\tIL\tDeKalb County\tH1\n60511\t17037\tBig rock\tIL\tDeKalb County\tH1\n60119\t17037\tElburn\tIL\tDeKalb County\tH1\n60145\t17037\tKingston\tIL\tDeKalb County\tH1\n60530\t17037\tLee\tIL\tDeKalb County\tH1\n60556\t17037\tWaterman\tIL\tDeKalb County\tH1\n60550\t17037\tShabbona\tIL\tDeKalb County\tH1\n60520\t17037\tHinckley\tIL\tDeKalb County\tH1\n60135\t17037\tGenoa\tIL\tDeKalb County\tH1\n60146\t17037\tKirkland\tIL\tDeKalb County\tH1\n60150\t17037\tMalta\tIL\tDeKalb County\tH1\n60518\t17037\tEarlville\tIL\tDeKalb County\tH1\n60140\t17037\tHampshire\tIL\tDeKalb County\tH1\n60151\t17037\tMaple park\tIL\tDeKalb County\tH1\n60129\t17037\tEsmond\tIL\tDeKalb County\tH1\n61735\t17039\tDewitt\tIL\tDe Witt County\tH1\n61745\t17039\tHeyworth\tIL\tDe Witt County\tH1\n61777\t17039\tWapella\tIL\tDe Witt County\tH1\n61750\t17039\tLane\tIL\tDe Witt County\tH1\n61756\t17039\tMaroa\tIL\tDe Witt County\tH1\n61839\t17039\tDe land\tIL\tDe Witt County\tH1\n61727\t17039\tClinton\tIL\tDe Witt County\tH1\n61754\t17039\tMc lean\tIL\tDe Witt County\tH1\n61882\t17039\tWeldon\tIL\tDe Witt County\tH1\n61778\t17039\tWaynesville\tIL\tDe Witt County\tH1\n61842\t17039\tFarmer city\tIL\tDe Witt County\tH1\n61752\t17039\tLe roy\tIL\tDe Witt County\tH1\n61749\t17039\tKenney\tIL\tDe Witt County\tH1\n62512\t17039\tBeason\tIL\tDe Witt County\tH1\n61872\t17041\tSadorus\tIL\tDouglas County\tH1\n61852\t17041\tLongview\tIL\tDouglas County\tH1\n61941\t17041\tMurdock\tIL\tDouglas County\tH1\n61851\t17041\tIvesdale\tIL\tDouglas County\tH1\n61956\t17041\tVilla grove\tIL\tDouglas County\tH1\n61913\t17041\tAtwood\tIL\tDouglas County\tH1\n61863\t17041\tPesotum\tIL\tDouglas County\tH1\n61943\t17041\tOakland\tIL\tDouglas County\tH1\n61911\t17041\tArthur\tIL\tDouglas County\tH1\n61919\t17041\tCamargo\tIL\tDouglas County\tH1\n61930\t17041\tHindsboro\tIL\tDouglas County\tH1\n61953\t17041\tTuscola\tIL\tDouglas County\tH1\n61910\t17041\tArcola\tIL\tDouglas County\tH1\n61917\t17041\tBrocton\tIL\tDouglas County\tH1\n61942\t17041\tNewman\tIL\tDouglas County\tH1\n60517\t17043\tWoodridge\tIL\tDuPage County\tH1\n60157\t17043\tMedinah\tIL\tDuPage County\tH1\n60172\t17043\tRoselle\tIL\tDuPage County\tH1\n60439\t17043\tLemont\tIL\tDuPage County\tH1\n60523\t17043\tOak brook\tIL\tDuPage County\tH1\n60502\t17043\tAurora\tIL\tDuPage County\tH1\n60143\t17043\tItasca\tIL\tDuPage County\tH1\n60555\t17043\tWarrenville\tIL\tDuPage County\tH1\n60559\t17043\tWestmont\tIL\tDuPage County\tH1\n60564\t17043\tNaperville\tIL\tDuPage County\tH1\n60540\t17043\tNaperville\tIL\tDuPage County\tH1\n60117\t17043\tBloomingdale\tIL\tDuPage County\tH1\n60514\t17043\tClarendon hills\tIL\tDuPage County\tH1\n60532\t17043\tLisle\tIL\tDuPage County\tH1\n60103\t17043\tBartlett\tIL\tDuPage County\tH1\n60106\t17043\tBensenville\tIL\tDuPage County\tH1\n60108\t17043\tBloomingdale\tIL\tDuPage County\tH1\n60599\t17043\tFox valley\tIL\tDuPage County\tH1\n60566\t17043\tNaperville\tIL\tDuPage County\tH1\n60187\t17043\tWheaton\tIL\tDuPage County\tH1\n60188\t17043\tCarol stream\tIL\tDuPage County\tH1\n60190\t17043\tWinfield\tIL\tDuPage County\tH1\n60567\t17043\tNaperville\tIL\tDuPage County\tH1\n60565\t17043\tNaperville\tIL\tDuPage County\tH1\n60522\t17043\tHinsdale\tIL\tDuPage County\tH1\n60598\t17043\tAurora\tIL\tDuPage County\tH1\n60189\t17043\tWheaton\tIL\tDuPage County\tH1\n60186\t17043\tWest chicago\tIL\tDuPage County\tH1\n60184\t17043\tWayne\tIL\tDuPage County\tH1\n60440\t17043\tBolingbrook\tIL\tDuPage County\tH1\n60120\t17043\tElgin\tIL\tDuPage County\tH1\n60137\t17043\tGlen ellyn\tIL\tDuPage County\tH1\n60007\t17043\tElk grove village\tIL\tDuPage County\tH1\n60181\t17043\tVilla park\tIL\tDuPage County\tH1\n60185\t17043\tWest chicago\tIL\tDuPage County\tH1\n60516\t17043\tDowners grove\tIL\tDuPage County\tH1\n60521\t17043\tHinsdale\tIL\tDuPage County\tH1\n60527\t17043\tWillowbrook\tIL\tDuPage County\tH1\n60139\t17043\tGlendale heights\tIL\tDuPage County\tH1\n60101\t17043\tAddison\tIL\tDuPage County\tH1\n60107\t17043\tStreamwood\tIL\tDuPage County\tH1\n60122\t17043\tCarol stream\tIL\tDuPage County\tH1\n60561\t17043\tDarien\tIL\tDuPage County\tH1\n60519\t17043\tEola\tIL\tDuPage County\tH1\n60193\t17043\tSchaumburg\tIL\tDuPage County\tH1\n60515\t17043\tDowners grove\tIL\tDuPage County\tH1\n60148\t17043\tLombard\tIL\tDuPage County\tH1\n60563\t17043\tNaperville\tIL\tDuPage County\tH1\n60569\t17043\tAurora\tIL\tDuPage County\tH1\n60191\t17043\tWood dale\tIL\tDuPage County\tH1\n60174\t17043\tSaint charles\tIL\tDuPage County\tH1\n60504\t17043\tAurora\tIL\tDuPage County\tH1\n60126\t17043\tElmhurst\tIL\tDuPage County\tH1\n60133\t17043\tHanover park\tIL\tDuPage County\tH1\n60138\t17043\tGlen ellyn\tIL\tDuPage County\tH1\n60199\t17043\tCarol stream\tIL\tDuPage County\tH1\n61933\t17045\tKansas\tIL\tEdgar County\tH1\n61955\t17045\tVermilion\tIL\tEdgar County\tH1\n61876\t17045\tSidell\tIL\tEdgar County\tH1\n61949\t17045\tRedmon\tIL\tEdgar County\tH1\n61850\t17045\tIndianola\tIL\tEdgar County\tH1\n61944\t17045\tParis\tIL\tEdgar County\tH1\n62441\t17045\tMarshall\tIL\tEdgar County\tH1\n61943\t17045\tOakland\tIL\tEdgar County\tH1\n61924\t17045\tChrisman\tIL\tEdgar County\tH1\n61810\t17045\tAllerton\tIL\tEdgar County\tH1\n61932\t17045\tHume\tIL\tEdgar County\tH1\n61917\t17045\tBrocton\tIL\tEdgar County\tH1\n61942\t17045\tNewman\tIL\tEdgar County\tH1\n61870\t17045\tRidge farm\tIL\tEdgar County\tH1\n62423\t17045\tDennison\tIL\tEdgar County\tH1\n61940\t17045\tMetcalf\tIL\tEdgar County\tH1\n62815\t17047\tBone gap\tIL\tEdwards County\tH1\n62844\t17047\tGrayville\tIL\tEdwards County\tH1\n62806\t17047\tAlbion\tIL\tEdwards County\tH1\n62833\t17047\tEllery\tIL\tEdwards County\tH1\n62818\t17047\tBrowns\tIL\tEdwards County\tH1\n62476\t17047\tWest salem\tIL\tEdwards County\tH1\n62479\t17049\tWheeler\tIL\tEffingham County\tH1\n62426\t17049\tEdgewood\tIL\tEffingham County\tH1\n62473\t17049\tWatson\tIL\tEffingham County\tH1\n62418\t17049\tBrownstown\tIL\tEffingham County\tH1\n62401\t17049\tEffingham\tIL\tEffingham County\tH1\n62414\t17049\tBeecher city\tIL\tEffingham County\tH1\n62838\t17049\tFarina\tIL\tEffingham County\tH1\n62411\t17049\tAltamont\tIL\tEffingham County\tH1\n62445\t17049\tMontrose\tIL\tEffingham County\tH1\n62443\t17049\tMason\tIL\tEffingham County\tH1\n62461\t17049\tShumway\tIL\tEffingham County\tH1\n62424\t17049\tDieterich\tIL\tEffingham County\tH1\n62880\t17049\tSaint peter\tIL\tEffingham County\tH1\n62444\t17049\tMode\tIL\tEffingham County\tH1\n62458\t17049\tSaint elmo\tIL\tEffingham County\tH1\n62462\t17049\tSigel\tIL\tEffingham County\tH1\n62467\t17049\tTeutopolis\tIL\tEffingham County\tH1\n62011\t17051\tBingham\tIL\tFayette County\tH1\n62885\t17051\tShobonier\tIL\tFayette County\tH1\n62471\t17051\tVandalia\tIL\tFayette County\tH1\n62892\t
